vi "Global_GenericIMAQCamera_HardwareConfig.vi"() -> ()   [LabVIEW 2011]
uses:
  GenericIMAQHardwareConfig.ctl
panel:
  in  "IMAQ Camera serial config":T1={"Use serial commands directly"=FALSE, "Frame rate set cmd"="ssf %d", "Exposure time set cmd"="set %d", "Frame rate get cmd"="get ssf", "Exposure time get cmd"="get set", "IMAQ Identifier"="img0", "Serial return skip chars"=2, "Set width/height"="get set", "Set offset xy"="get set", "Get width"="get set", "Get height"="get set", "Get offset X"="get set", "Get offset Y"="get set"}
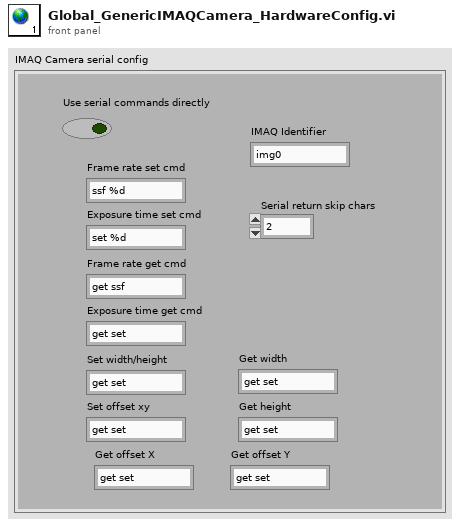
[diagram p1: front panel]
types:
  T1 = typedef "GenericIMAQHardwareConfig.ctl" = cluster{"Use serial commands directly":bool, "Frame rate set cmd":string, "Exposure time set cmd":string, "Frame rate get cmd":string, "Exposure time get cmd":string, "IMAQ Identifier":string, "Serial return skip chars":i32, "Set width/height":string, "Set offset xy":string, "Get width":string, "Get height":string, "Get offset X":string, "Get offset Y":string}
diagram:
